vi "DMA.Write.vi"   [LabVIEW 2016, in "GE 5565PIORC.lvclass"]
uses:
  GE 5565PIORC.lvclass
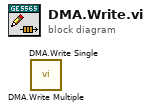
[diagram p0: block diagram]
diagram:
  n1 = call "DMA.Write Multiple.vi"() -> ()  [unwired: 8 in, 4 out]
  n2 = call "DMA.Write Single.vi"() -> ()  [unwired: 8 in, 4 out]
